vi "Load Image (UTF-8 Path).vi"(8 "error in (no error)":errorcluster, 9 "Transparency Threshold (127)":u8=127, 11 "Path In":string) -> (0 "error out":errorcluster, 2 "Image":T1, 3 "Path Out":string)   [LabVIEW 2020, in "G-Image.lvlib"]
doc: "Load an image file from disk, and return it as a LabVIEW picture."
uses:
  G-Image.lvlib
  <vilib>/picture/picture.llb/imagedata.ctl
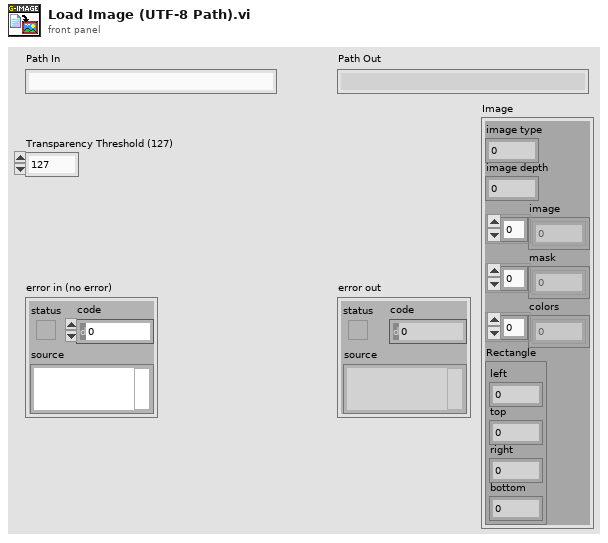
[diagram p1: front panel]
types:
  T1 = typedef "imagedata.ctl" = cluster{"image type":i32, "image depth":i32, "image":u8[], "mask":u8[], "colors":u32[], "Rectangle":cluster{"left":i16, "top":i16, "right":i16, "bottom":i16}}
  T2 = typedef "G-Image.lvlib/Extended Image.ctl" = cluster{"Image":T1, "Layers":i32, "Delays":i32[]}
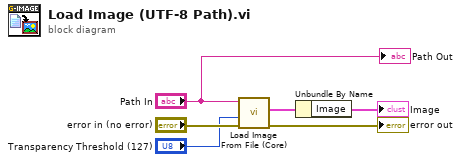
[diagram p0: block diagram]
diagram:
  n1 = call "Load Image From File (Core).vi"("error in (no error)"="error in (no error)", "Transparency Threshold (127)"="Transparency Threshold (127)", "Path In"="Path In") -> ("error out"=→"error out":errorcluster, "Extended Image"=w3:T2)  [unwired: 6 in, 1 out]
  n2 = Unbundle By Name(w3) -> ("Image"=→"Image":T1)
  "Path Out" <- "Path In"
